vi "Get Shared Variables.vi"(8 "error in (no error)":errorcluster, 11 "IP Address":string) -> ()   [LabVIEW 2012, in "Shared Variable Custom Device.lvlib"]
uses:
  Shared Variable Custom Device.lvlib
  Shared Variable Data.ctl
  <vilib>/Utility/VariantDataType/Type.ctl
  Shared/Shared Variable Globals.vi
  <resource>/objmgr/ni.var.rc
  <vilib>/Utility/VariantDataType/VariantType.lvlib
panel:
  out "Array":T1[](array[typedef])
  in  "Previous Button":bool
  in  "Next Button":bool
  in  "VeriStand Tree":string[](tree)
  in  "Stop Button":bool
  in  "Shared Variable Tree":string[](tree)
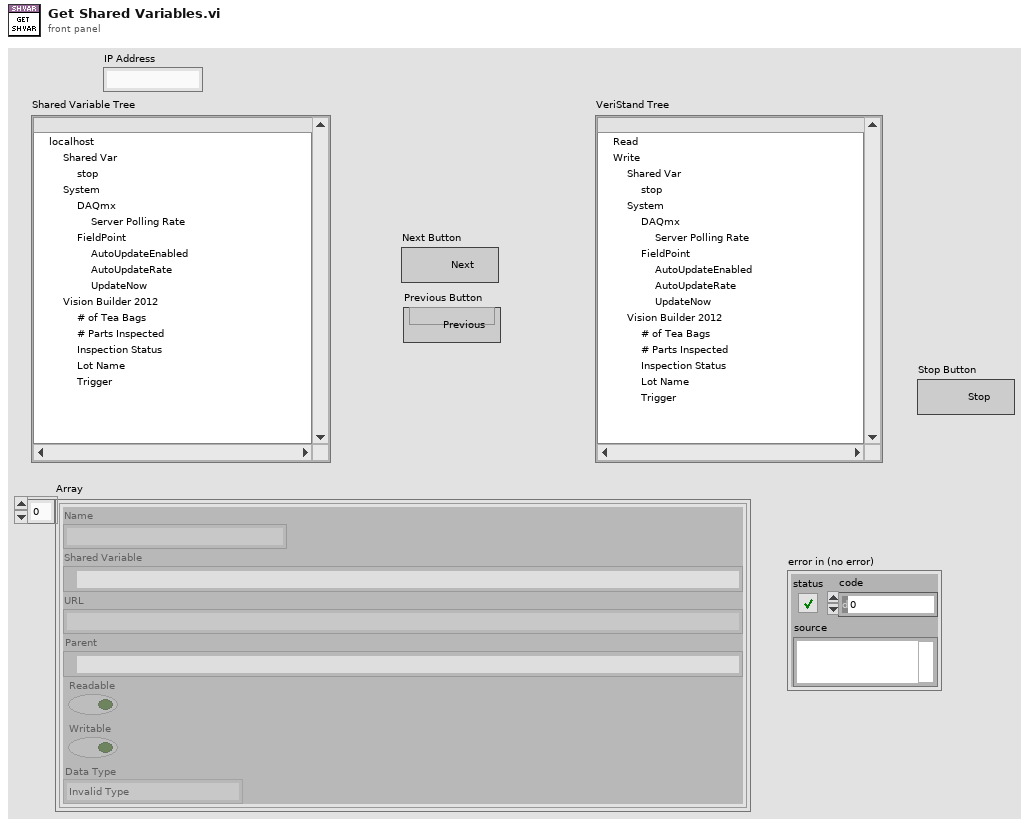
[diagram p1: front panel]
types:
  T1 = typedef "Shared Variable Custom Device.lvlib/Shared Variable Data.ctl" = cluster{"Name":string, "Shared Variable":refnum<k21>, "URL":string, "Parent":refnum<k21>, "Readable":bool, "Writable":bool, "Data Type":T2}
  T2 = typedef "VariantType.lvlib/Type.ctl" = enum8{"Invalid Type", "Void", "I8", "I16", "I32", "I64", "U8", "U16", "U32", "U64", "Single Float", "Double Float", "Extended Float", "Single Complex", "Double Complex", "Extended Complex", "Enum U8", "Enum U16", "Enum U32", "Enum U64", "Single Float With Unit", "Double Float With Unit", "Extended Float With Unit", "Single Complex with Unit", "Double Complex with Unit", "Extended Complex with Unit", "Boolean", "String", "Path", "Picture", "Tag", "Array", "Cluster", "Variant", "LV Variant", "Waveform", "Timestamp", "Digital Waveform", "Digital Data", "ExpressData", "Refnum", "External Data", "VI", "Poly VI", "LabVIEW Class Instance", "Fixed Point"}
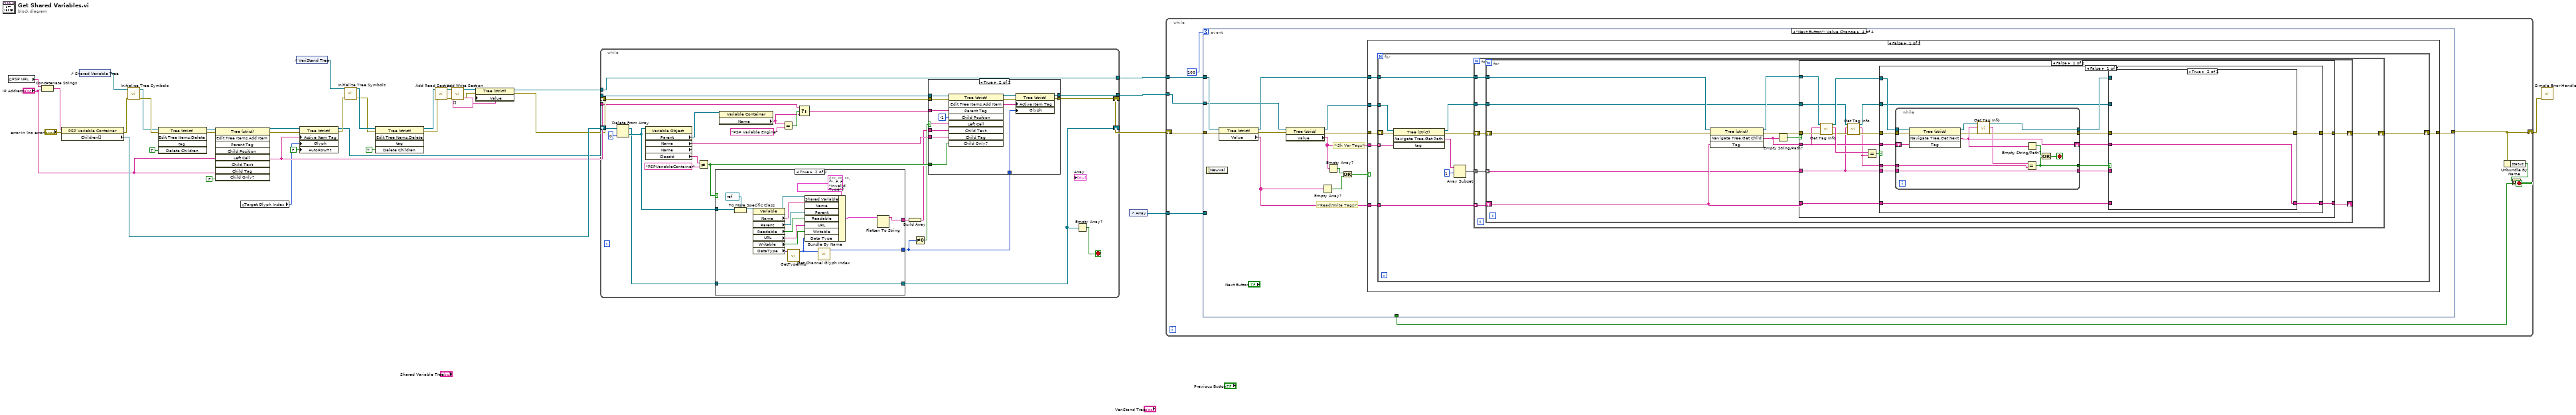
[diagram p0: block diagram]
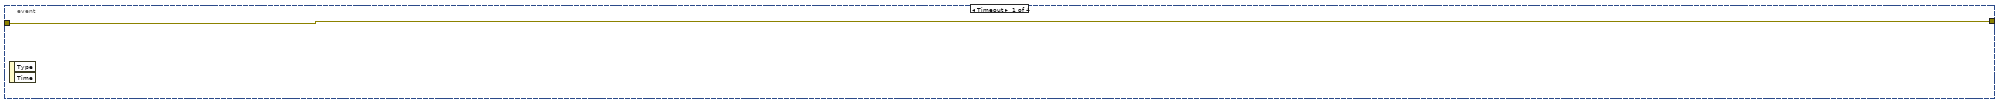
[diagram p2: hidden frame]
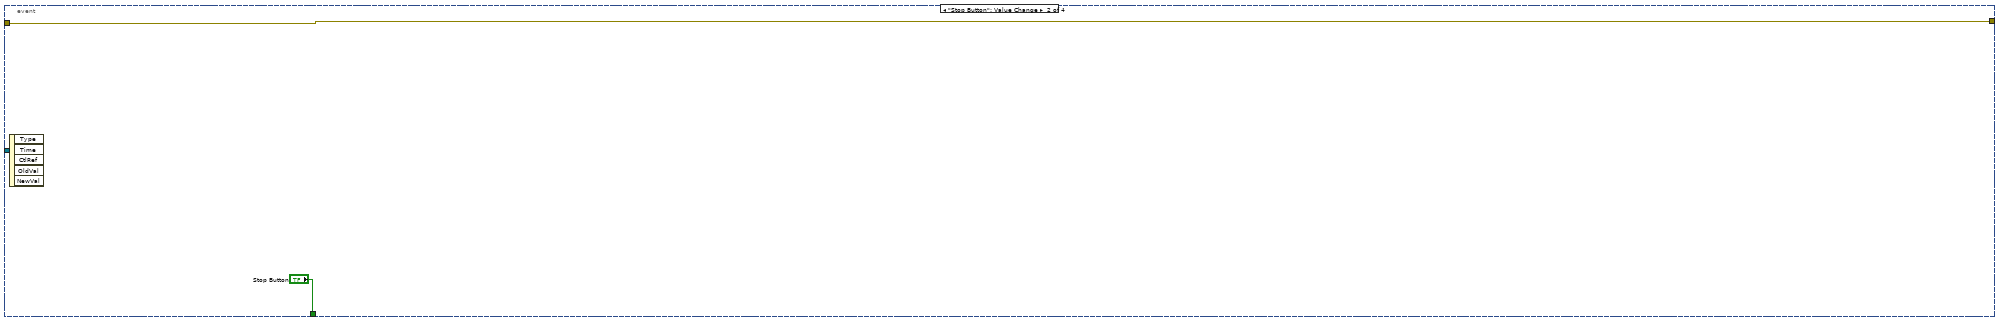
[diagram p3: hidden frame]
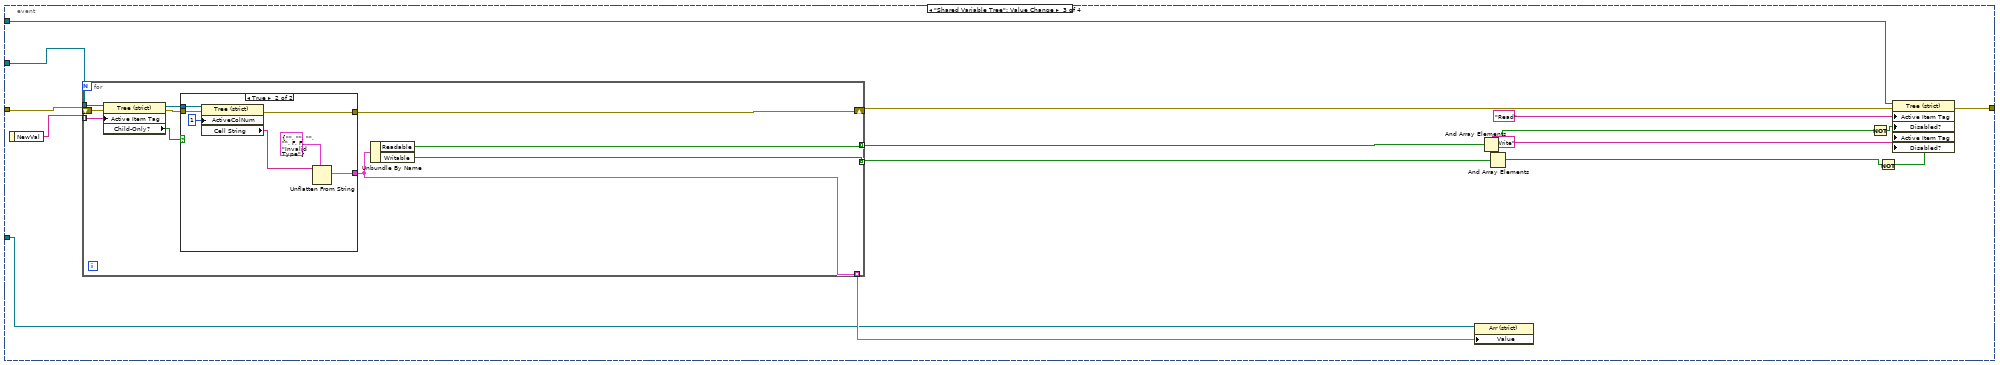
[diagram p4: hidden frame]
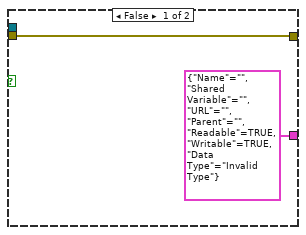
[diagram p5: hidden frame]
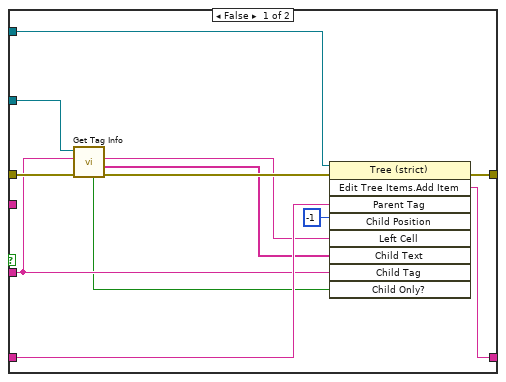
[diagram p6: hidden frame]
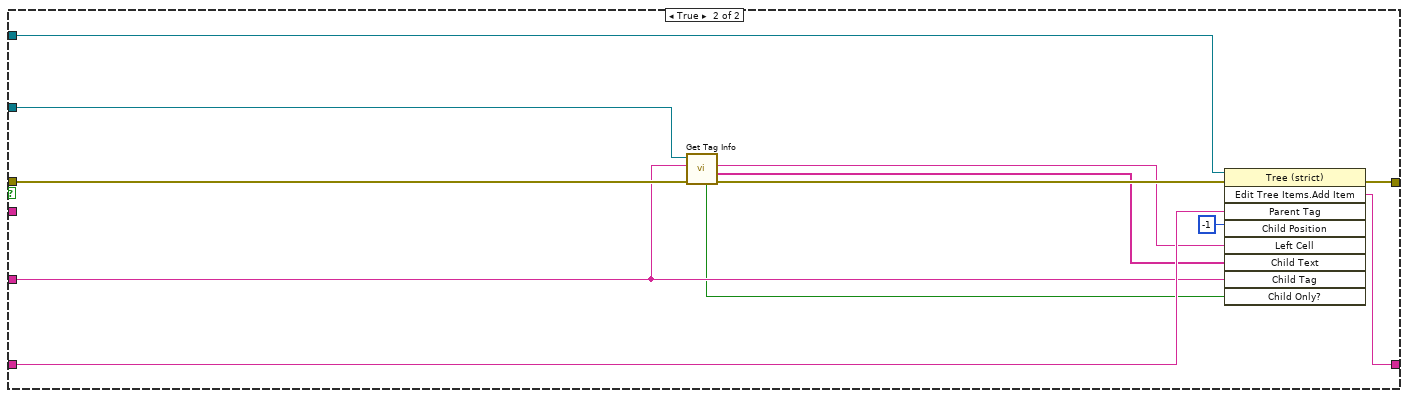
[diagram p8: hidden frame]
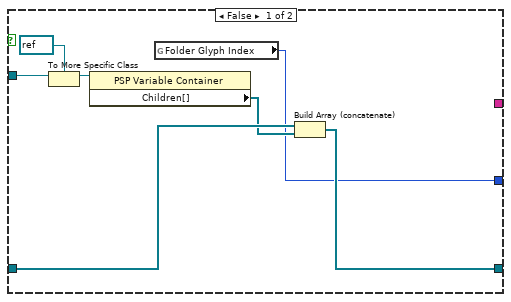
[diagram p11: hidden frame]
diagram:
  n1 = global read "Shared Variable Globals.vi" "PSP URL"() -> (w38:string)
  n2 = Concatenate Strings(w38, "IP Address") -> (w36:string)
  n3 = property class="PSP Variable Container"(reference=w36, error in="error in (no error)") -> (error out=w29:errorcluster, "Children[]"=w35:refnum<k21>[])  [unwired: 1 out]
  n4 = control-ref of="Shared Variable Tree"() -> (w27:refnum<vi>)
  n5 = call "Initialize Tree Symbols.vi"("error in (no error)"=w29, "TreeControl in"=w27) -> ("error out"=w28:errorcluster, "TreeControl out"=w26:refnum<vi>)  [unwired: 8 in]
  n6 = invoke class="Tree (strict)" method="Edit Tree Items.Delete"(reference=w26, error in=w28, "Delete Children"=TRUE ("Delete Children?")) -> (reference out=w31:refnum<vi>, error out=w32:errorcluster)  [unwired: 2 in, 3 out]
  n7 = invoke class="Tree (strict)" method="Edit Tree Items.Add Item"(reference=w31, error in=w32, "Left Cell"="IP Address", "Child Tag"="IP Address", "Child Only?"=FALSE) -> (reference out=w24:refnum<vi>, error out=w25:errorcluster, "Edit Tree Items:Add Item"=w23:string)  [unwired: 4 in, 6 out]
  n8 = global read "Shared Variable Globals.vi" "Target Glyph Index"() -> (w22:i32)
  n9 = control-ref of="VeriStand Tree"() -> (w14:refnum<vi>)
  n10 = property class="Tree (strict)"(reference=w24, error in=w25, "Active Item Tag"=w23, "Glyph"=w22, "AutoRowHt"=FALSE ("Autosizing Row Height")) -> (reference out=w15:refnum<vi>, error out=w16:errorcluster)
  n11 = call "Initialize Tree Symbols.vi"("error in (no error)"=w16, "TreeControl in"=w14) -> ("error out"=w18:errorcluster, "TreeControl out"=w19:refnum<vi>)  [unwired: 8 in]
  n12 = invoke class="Tree (strict)" method="Edit Tree Items.Delete"(reference=w19, error in=w18, "Delete Children"=TRUE ("Delete Children?")) -> (reference out=w11:refnum<vi>, error out=w12:errorcluster)  [unwired: 2 in, 3 out]
  n13 = call "Add Read Section.vi"("error in (no error)"=w12, "TreeControl in"=w11) -> ("error out"=w13:errorcluster, "TreeControl out"=w10:refnum<vi>)  [unwired: 7 in, 1 out]
  n14 = call "Add Write Section.vi"("error in (no error)"=w13, "TreeControl in"=w10) -> ("error out"=w7:errorcluster, "TreeControl out"=w8:refnum<vi>)  [unwired: 7 in, 1 out]
  n15 = property class="Tree (strict)"(reference=w8, error in=w7, "Value"=string[] []) -> (reference out=w5:refnum<vi>, error out=w6:errorcluster)
  n16 = while {
    tunnel: w15 -> [w62]
    tunnel: w23 -> [w51]
    shift-right: [w45] -> w21
    shift-left: w6 -> [w63]
    shift-right: [w54] -> _
    shift-left: w35 -> [w59]
    tunnel: [w40] -> w3
    tunnel: w5 -> [w39]
    tunnel: [w39] -> w2
    stop <- w61 stop-if-true
    n17 = Delete From Array(array=w59, index=0) -> (deleted portion=w56:refnum<k21>, array with subset deleted=w55:refnum<k21>[])  [unwired: 1 in]
    n18 = property class="Variable Object" props=["Parent", "Name", "Name", "ClassId"](reference=w56) -> ("Parent"=w47:refnum<k21>, "Name"=w46:string, "ClassId"=w48:string)  [unwired: 1 in, 3 out]
    n19 = Not Equal?(x=w48, y="PSPVariableContainer" ("Name")) -> (x != y?=w57:bool)
    n20 = case shown="True" w57 {
      tunnel: w56 -> [w85 w100]
      tunnel: w55 -> [w82 w101]
      tunnel: [w80 w101] -> w54
      tunnel: [w79 w97] -> w44
      tunnel: [_ w86] -> w42
      frame False {
        n21 = To More Specific Class(target class=refnum<k21> refnum ("Local PSP Variable Root Container"), reference=w85) -> (specific class reference=w83:refnum<k21>)  [unwired: 1 in, 1 out]
        n22 = property class="PSP Variable Container"(reference=w83) -> ("Children[]"=w81:refnum<k21>[])  [unwired: 1 in, 2 out]
        n23 = global read "Shared Variable Globals.vi" "Folder Glyph Index"() -> (w79:i32)
        n24 = Build Array (concatenate)(w82, w81) -> (w80:refnum<k21>[])
      }
      frame True {
        n25 = To More Specific Class(target class=refnum<k21> refnum ("Root"), reference=w100) -> (specific class reference=w98:refnum<k21>)  [unwired: 1 in, 1 out]
        n26 = property class="Variable"(reference=w98) -> (reference out=w94:refnum<k21>, "Name"=w93:string, "Parent"=w92:refnum<k21>, "Readable"=w91:bool, "URL"=w90:string, "Writable"=w89:bool, "DataType"=w96:variant)  [unwired: 1 in, 1 out]
        n27 = call <vilib>:"GetTypeInfo.vi"("Variant"=w96) -> ("Type Enum"=w88:T2)  [unwired: 6 in, 4 out]
        n28 = Bundle By Name(cluster=T1 {"Name"="", "Shared Variable"="", "URL"="", "Parent"="", "Readable"=FALSE, "Writable"=FALSE, "Data Type"=enum."Invalid Type"} ("Shared Variable Data"), "Shared Variable"=w94, "Name"=w93, "Parent"=w92, "Readable"=w91, "URL"=w90, "Writable"=w89, "Data Type"=w88) -> (w87:T1)
        n29 = call "Get Channel Glyph Index.vi"("Channel Type"=w88) -> ("Glyph Index"=w97:i32)  [unwired: 10 in]
        n30 = Flatten To String(anything=w87) -> (data string=w86:string)  [unwired: 3 in, 2 out]
      }
    }
    n31 = property class="Variable Container"(reference=w47) -> ("Name"=w50:string)  [unwired: 1 in, 2 out]
    n32 = Equal?(x=w50, y="PSP Variable Engine" ("Name")) -> (x = y?=w52:bool)
    n33 = Select(t=w51, s=w52, f=w50) -> (s? t:f=w49:string)
    n34 = Build Array(w42) -> (w41:string[])
    n35 = Not Equal To 0?(x=w44) -> (x != 0?=w43:bool)
    n36 = case shown="True" w43 {
      tunnel: w63 -> [w65 w78]
      tunnel: w62 -> [w64 w77]
      tunnel: w57 -> [_ w75]
      tunnel: w49 -> [_ w74]
      tunnel: w46 -> [_ w73]
      tunnel: [w65 w70] -> w45
      tunnel: w44 -> [_ w68]
      tunnel: w41 -> [_ w67]
      tunnel: [w64 w66] -> w40
      frame False {
      }
      frame True {
        n37 = invoke class="Tree (strict)" method="Edit Tree Items.Add Item"(reference=w77, error in=w78, "Parent Tag"=w74, "Child Position"=-1, "Left Cell"=w73, "Child Text"=w67, "Child Tag"=w73, "Child Only?"=w75) -> (reference out=w71:refnum<vi>, error out=w72:errorcluster, "Edit Tree Items:Add Item"=w69:string)  [unwired: 1 in, 6 out]
        n38 = property class="Tree (strict)"(reference=w71, error in=w72, "Active Item Tag"=w69, "Glyph"=w68) -> (reference out=w66:refnum<vi>, error out=w70:errorcluster)
      }
    }
    n39 = Empty Array?(array=w54) -> (empty?=w61:bool)
  }
  n40 = control-ref of="Array"() -> (w9:refnum<vi>)
  n41 = while {
    tunnel: w3 -> [w108]
    shift-right: [w106] -> w1
    shift-left: w21 -> [w109]
    tunnel: w2 -> [w102]
    tunnel: w9 -> [w107]
    stop <- w103 stop-if-true
    n42 = event shown="[3] \"Next Button\": Value Change" {
      selector: _ -> [_ _ _ _]
      dyn-events: _ -> [_ _ _ _]
      timeout: 100 ("Numeric") -> [_ _ _ _]
      tunnel: [_ "Stop Button" _ _] -> w105
      tunnel: w109 -> [w111 w112 w128 w151]
      tunnel: [w111 w112 w121 w156] -> w106
      tunnel: w108 -> [_ _ w127 w159]
      tunnel: w107 -> [_ _ w124 _]
      tunnel: w102 -> [_ _ w120 w160]
      event Timeout {
        n43 = event-data() -> ()  [unwired: 1 in, 2 out]
      }
      event "Stop Button": Value Change {
        n44 = event-data() -> ()  [unwired: 1 in, 5 out]
      }
      event "Shared Variable Tree": Value Change {
        n45 = event-data() -> ("NewVal"=w126:string[])  [unwired: 1 in]
        n46 = for {
          tunnel: w127 -> [w136]
          shift-right: [w138] -> w121
          shift-left: w128 -> [w137]
          tunnel: w126 -> [w132] mode=indexing
          tunnel: [w131] -> w125 mode=indexing
          tunnel: [w130] -> w122 mode=indexing
          tunnel: [w129] -> w123 mode=indexing
          n47 = property class="Tree (strict)"(reference=w136, error in=w137, "Active Item Tag"=w132) -> (reference out=w134:refnum<vi>, error out=w135:errorcluster, "Child-Only?"=w133:bool)
          n48 = case shown="True" w133 {
            tunnel: [w140 w146] -> w138
            tunnel: w135 -> [w140 w145]
            tunnel: w134 -> [_ w144]
            tunnel: [T1 {"Name"="", "Shared Variable"="", "URL"="", "Parent"="", "Readable"=TRUE, "Writable"=TRUE, "Data Type"=enum."Invalid Type"} ("Shared Variable Data") w141] -> w131
            frame False {
            }
            frame True {
              n49 = property class="Tree (strict)"(reference=w144, error in=w145, "ActiveColNum"=1 ("Active Cell:Active Column Number")) -> (error out=w146:errorcluster, "Cell String"=w143:string)  [unwired: 1 out]
              n50 = Unflatten From String(type=T1 {"Name"="", "Shared Variable"="", "URL"="", "Parent"="", "Readable"=FALSE, "Writable"=FALSE, "Data Type"=enum."Invalid Type"} ("Shared Variable Data"), binary string=w143) -> (value=w141:T1)  [unwired: 3 in, 2 out]
            }
          }
          n51 = Unbundle By Name(w131) -> ("Readable"=w130:bool, "Writable"=w129:bool)
        }
        n52 = property class="Arr (strict)"(reference=w124, "Value"=w125) -> ()  [unwired: 1 in, 2 out]
        n53 = And Array Elements(Boolean array=w122) -> (logical AND=w118:bool)
        n54 = And Array Elements(Boolean array=w123) -> (logical AND=w115:bool)
        n55 = Not(x=w118) -> (.not. x?=w117:bool)
        n56 = Not(x=w115) -> (.not. x?=w114:bool)
        n57 = property class="Tree (strict)"(reference=w120, error in=w121, "Active Item Tag"="Read" ("Active Item:Tag"), "Disabled?"=w117, "Active Item Tag"="Write" ("Active Item:Tag"), "Disabled?"=w114) -> ()  [unwired: 2 out]
      }
      event "Next Button": Value Change {
        # ">Sh Var Tags>"
        # ">Read/Write Tags>"
        n58 = event-data() -> ()  [unwired: 1 in, 1 out]
        n59 = property class="Tree (strict)"(reference=w160, error in=w151) -> (reference out=w154:refnum<vi>, error out=w150:errorcluster, "Value"=w153:string[])
        n60 = property class="Tree (strict)"(reference=w159, error in=w150) -> (reference out=w155:refnum<vi>, error out=w152:errorcluster, "Value"=w157:string[])
        n61 = Empty Array?(array=w153) -> (empty?=w148:bool)
        n62 = Empty Array?(array=w157) -> (empty?=w149:bool)
        n63 = Or(x=w149, y=w148) -> (x .or. y?=w158:bool)
        n64 = case shown="False" w158 {
          tunnel: w157 -> [w164 _]
          tunnel: w152 -> [w166 w266]
          tunnel: w155 -> [w165 _]
          tunnel: [w163 w266] -> w156
          tunnel: w154 -> [w162 _]
          tunnel: w153 -> [w161 _]
          frame False {
            n65 = for {
              tunnel: w165 -> [w177]
              shift-right: [w170] -> w163
              shift-left: w166 -> [w168]
              tunnel: w164 -> [w176] mode=indexing
              tunnel: w162 -> [w175]
              tunnel: w161 -> [w169]
              n66 = invoke class="Tree (strict)" method="Navigate Tree.Get Path"(reference=w177, error in=w168, "tag"=w176) -> (reference out=w167:refnum<vi>, error out=w171:errorcluster, "Navigate Tree:Get Path"=w173:string[])  [unwired: 1 in, 1 out]
              n67 = Array Subset(array=w173, index=1) -> (w172:string[])  [unwired: 1 in]
              n68 = for {
                tunnel: w175 -> [w183]
                tunnel: w169 -> [w180] mode=indexing
                shift-right: [w181] -> w170
                shift-left: w171 -> [w182]
                tunnel: w172 -> [w179]
                tunnel: w167 -> [w178]
                n69 = for {
                  tunnel: w183 -> [w194]
                  tunnel: w179 -> [w186] mode=indexing
                  shift-right: [w192] -> w181
                  shift-left: w182 -> [w193]
                  shift-right: [w187] -> _
                  shift-left: w180 -> [w191]
                  tunnel: w178 -> [w184]
                  n70 = invoke class="Tree (strict)" method="Navigate Tree.Get Child"(reference=w194, error in=w193, "Tag"=w191) -> (reference out=w189:refnum<vi>, error out=w185:errorcluster, "Navigate Tree:Get Child"=w188:string)  [unwired: 1 in, 1 out]
                  n71 = Empty String/Path?(string/path=w188) -> (empty?=w190:bool)
                  n72 = case shown="False" w190 {
                    tunnel: [w208 w264] -> w192
                    tunnel: w191 -> [w207 w263]
                    tunnel: w186 -> [w196 w258]
                    tunnel: w185 -> [w205 w260]
                    tunnel: w189 -> [w204 w262]
                    tunnel: w188 -> [w202 _]
                    tunnel: [w206 w261] -> w187
                    tunnel: w184 -> [w198 w259]
                    frame False {
                      n73 = call "Get Tag Info.vi"("error in (no error)"=w205, "Tag"=w202, "TreeControl in"=w204) -> ("error out"=w201:errorcluster, "Left Cell String"=w203:string, "TreeControl out"=w199:refnum<vi>)  [unwired: 4 in, 2 out]
                      n74 = call "Get Tag Info.vi"("error in (no error)"=w201, "Tag"=w196, "TreeControl in"=w198) -> ("error out"=w200:errorcluster, "Left Cell String"=w195:string, "TreeControl out"=w197:refnum<vi>)  [unwired: 4 in, 2 out]
                      n75 = Equal?(x=w203, y=w195) -> (x = y?=w209:bool)
                      n76 = case shown="False" w209 {
                        tunnel: w200 -> [w223 w253]
                        tunnel: [w219 w253] -> w208
                        tunnel: w199 -> [w222 _]
                        tunnel: w202 -> [w221 w252]
                        tunnel: w196 -> [w216 _]
                        tunnel: w207 -> [w217 _]
                        tunnel: [w215 w252] -> w206
                        tunnel: w197 -> [w213 _]
                        tunnel: w195 -> [w211 _]
                        frame False {
                          n77 = while {
                            tunnel: w223 -> [w251]
                            tunnel: w222 -> [w250]
                            shift-right: [w240] -> w210
                            shift-left: w221 -> [w249]
                            tunnel: w216 -> [w245]
                            tunnel: [w241] -> w220
                            tunnel: [w242] -> w218
                            tunnel: [w246] -> w214
                            tunnel: [w245] -> w212
                            tunnel: w211 -> [w238]
                            stop <- w248 stop-if-true
                            n78 = invoke class="Tree (strict)" method="Navigate Tree.Get Next"(reference=w250, error in=w251, "Tag"=w249) -> (reference out=w243:refnum<vi>, error out=w244:errorcluster, "Navigate Tree:Get Next Item"=w240:string)  [unwired: 1 in, 1 out]
                            n79 = call "Get Tag Info.vi"("error in (no error)"=w244, "Tag"=w240, "TreeControl in"=w243) -> ("error out"=w241:errorcluster, "Left Cell String"=w239:string, "TreeControl out"=w242:refnum<vi>)  [unwired: 4 in, 2 out]
                            n80 = Equal?(x=w239, y=w238) -> (x = y?=w246:bool)
                            n81 = Empty String/Path?(string/path=w240) -> (empty?=w247:bool)
                            n82 = Or(x=w247, y=w246) -> (x .or. y?=w248:bool)
                          }
                          n83 = case shown="True" w214 {
                            tunnel: w220 -> [w231 w237]
                            tunnel: [w234 w237] -> w219
                            tunnel: w218 -> [w228 _]
                            tunnel: w217 -> [w233 _]
                            tunnel: [w232 w236] -> w215
                            tunnel: w213 -> [w230 _]
                            tunnel: w212 -> [w225 _]
                            tunnel: w210 -> [_ w236]
                            frame False {
                              n84 = call "Get Tag Info.vi"("error in (no error)"=w231, "Tag"=w225, "TreeControl in"=w230) -> ("error out"=w229:errorcluster, "Child Text"=w226:string[], "Left Cell String"=w227:string, "Child-Only?"=w224:bool)  [unwired: 4 in, 1 out]
                              n85 = invoke class="Tree (strict)" method="Edit Tree Items.Add Item"(reference=w228, error in=w229, "Parent Tag"=w233, "Child Position"=-1, "Left Cell"=w227, "Child Text"=w226, "Child Tag"=w225, "Child Only?"=w224) -> (error out=w234:errorcluster, "Edit Tree Items:Add Item"=w232:string)  [unwired: 1 in, 7 out]
                            }
                            frame True {
                            }
                          }
                        }
                        frame True {
                        }
                      }
                    }
                    frame True {
                      n86 = call "Get Tag Info.vi"("error in (no error)"=w260, "Tag"=w258, "TreeControl in"=w259) -> ("error out"=w257:errorcluster, "Child Text"=w255:string[], "Left Cell String"=w256:string, "Child-Only?"=w254:bool)  [unwired: 4 in, 1 out]
                      n87 = invoke class="Tree (strict)" method="Edit Tree Items.Add Item"(reference=w262, error in=w257, "Parent Tag"=w263, "Child Position"=-1, "Left Cell"=w256, "Child Text"=w255, "Child Tag"=w258, "Child Only?"=w254) -> (error out=w264:errorcluster, "Edit Tree Items:Add Item"=w261:string)  [unwired: 1 in, 7 out]
                    }
                  }
                }
              }
            }
          }
          frame True {
          }
        }
      }
    }
    n88 = Unbundle By Name(w106) -> ("status"=w104:bool)
    n89 = Or(x=w104, y=w105) -> (x .or. y?=w103:bool)
  }
  n90 = call <vilib>:"Simple Error Handler.vi"("error in (no error)"=w1) -> ()  [unwired: 4 in, 5 out]
